vi "Calculate Mean of Section.vi"(9 "# of Samples Averaged\nfor standing weight\n(500 is default)":i32, 10 "Start of Sample":dbl, 11 "Dynamic Data Type":dynamicdata(waveform)) -> (3 "Average":dynamicdata(waveform))   [LabVIEW 2016]
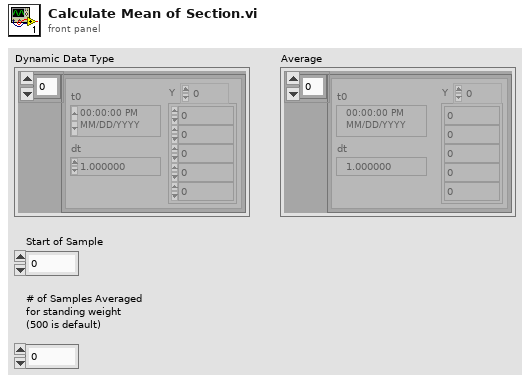
[diagram p1: front panel]
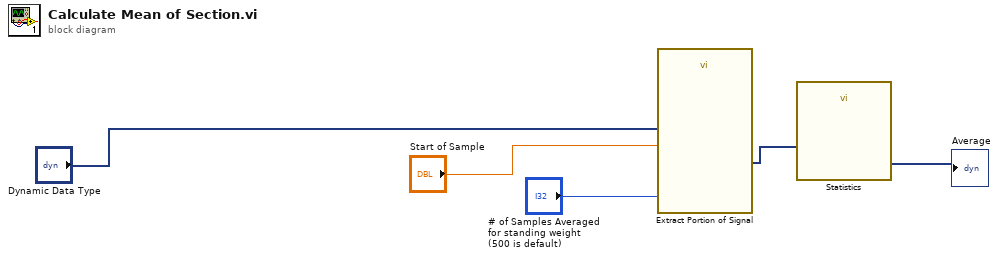
[diagram p0: block diagram]
diagram:
  n1 = call "Extract Portion of Signal"("Samples"="# of Samples Averaged\nfor standing weight\n(500 is default)", "Begin Sample"="Start of Sample", "Signals"="Dynamic Data Type") -> ("Section"=w1:dynamicdata)  [unwired: 7 in, 1 out]
  n2 = call "Statistics"("Signals"=w1) -> ("Arithmetic Mean"=→"Average":dynamicdata)  [unwired: 25 in, 1 out]
